vi "AgPSA _Set Up Zspan.vi"(6 "Manual Attenuation (dB)":dbl=30.0, 8 "error in (no error)":errorcluster, 9 "Reference Level (dBm)":dbl=20.0, 10 "Sweep Points":u32=8192, 11 "VISA Refnum in":refnum<visa-resource-name>) -> (0 "error out":errorcluster, 3 "VISA Refnum out":refnum<visa-resource-name>)   [LabVIEW 2015]
uses:
  <instrlib>/Agilent ESA PSA Series/Agilent ESA PSA Series.lvlib
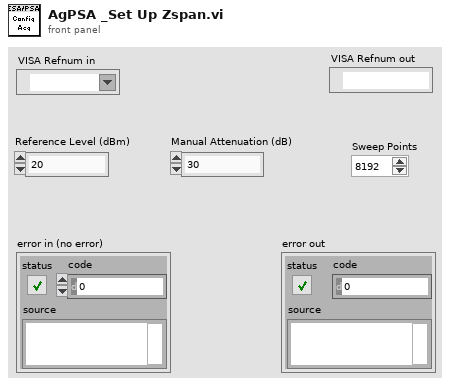
[diagram p1: front panel]
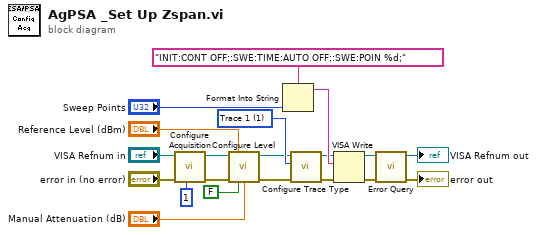
[diagram p0: block diagram]
diagram:
  w8 = u16 1 items=["Trace 1"=1, "Trace 2"=2, "Trace 3"=3] ("Trace Name (1: Trace 1)")
  n1 = call <instrlib>:"Configure Acquisition.vi"("Vertical Scale (0: Linear)"=1, "error in (no error)"="error in (no error)", "VISA resource name"="VISA Refnum in") -> ("error out"=w15:errorcluster, "VISA resource name out"=w17:refnum<visa-resource-name>)  [unwired: 7 in]
  n2 = call "Configure Level.vi"("VISA resource name"=w17, "Reference Level (dBm)"="Reference Level (dBm)", "error in (no error)"=w15, "Enable Auto Attenuation"=FALSE ("Enable Auto Attenuation (T: Enable)"), "Manual Attenuation (dB)"="Manual Attenuation (dB)") -> ("VISA resource name out"=w6:refnum<visa-resource-name>, "error out"=w5:errorcluster)  [unwired: 9 in]
  n3 = Format Into String(format string="INIT:CONT OFF;:SWE:TIME:AUTO OFF;:SWE:POIN %d;", "Sweep Points") -> (resulting string=w13:string)  [unwired: 2 in, 1 out]
  n4 = call <instrlib>:"Configure Trace Type.vi"("error in (no error)"=w5, "Trace Name (1: Trace 1)"=w8, "VISA resource name"=w6) -> ("error out"=w9:errorcluster, "VISA resource name out"=w10:refnum<visa-resource-name>)  [unwired: 7 in]
  n5 = VISA Write(VISA resource name=w10, write buffer=w13, error in (no error)=w9) -> (VISA resource name out=w11:refnum<visa-resource-name>, error out=w12:errorcluster)  [unwired: 1 out]
  n6 = call <instrlib>:"Error Query.vi"("error in (no error)"=w12, "VISA resource name"=w11) -> ("error out"=→"error out":errorcluster, "VISA resource name out"=→"VISA Refnum out":refnum<visa-resource-name>)  [unwired: 6 in, 2 out]
